vi "Driver Init.vi"(8 "error in (no error)":errorcluster, 11 "MSX-E3701 in":refnum<class "MSX-E3701.lvclass">) -> (0 "error out":errorcluster, 3 "MSX-E3701 out":refnum<class "MSX-E3701.lvclass">)   [LabVIEW 2014, in "MSX-E3701.lvlib" / "MSX-E3701.lvclass"]
doc: "Inicializa los valores recomendados por el datasheet del ADDI-DATA para iniciar la adquisición de datos en cualquiera de sus modos. Ademas inicia Los valores del Diagnostic, ganancia y offset."
uses:
  MSX-E3701.lvclass
  API/Typedef/Diagnostic Data.ctl
  MSX-E3701.lvclass/MSX-E3701.ctl
  DriverMasterSync/build/DriverMasterSync.lvlibp/Modules/HAL/DriverMasterSync/DriverMasterSyncClass/DriverMasterSync.lvclass
  API/MSX-E3701_dll.lvlib
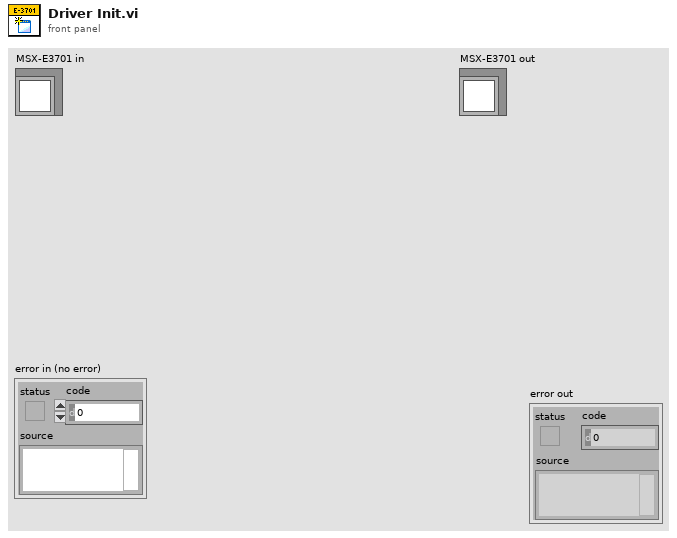
[diagram p1: front panel]
types:
  T1 = typedef "MSX-E3701_dll.lvlib/Diagnostic Data.ctl" = cluster{"Muestras Diag. Cycle":u32, "Tolerancia Cycle":sgl, "Tolerancia":sgl, "Mask Proteccion T":u64, "Promedio Transd":sgl[]}
  T2 = typedef "DriverMasterSync.lvlibp/HAL Config Data.ctl" = cluster{"HWSync Index":u32, "Driver Name":string, "Channel Mask":u64}
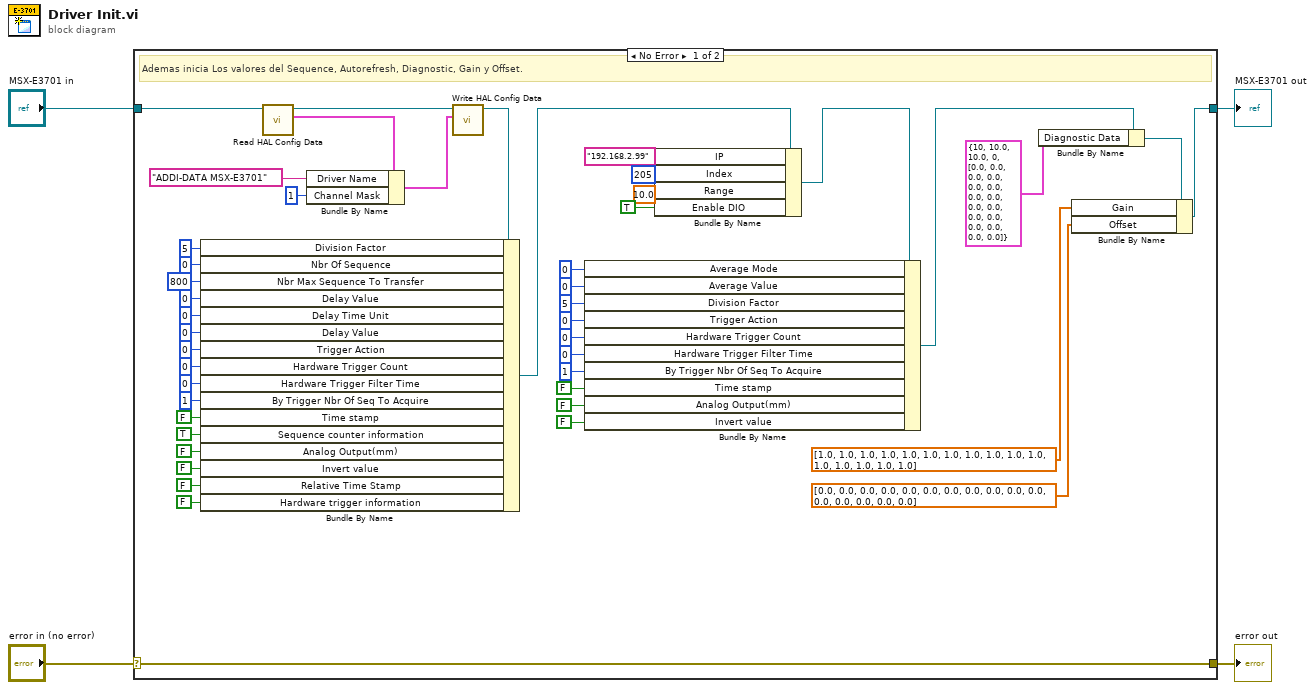
[diagram p0: block diagram]
diagram:
  n1 = case shown="No Error" "error in (no error)" {
    selector: "error in (no error)" -> [w50 w52]
    tunnel: [w50 w52] -> w3
    tunnel: [w16 w51] -> w1
    tunnel: "MSX-E3701 in" -> [w48 w51]
    frame No Error {
      # "Ademas inicia Los valores del Sequence, Autorefresh, Diagnostic, Gain y Offset."
      n2 = call "Read HAL Config Data.vi"("DriverMasterSync in"=w48) -> ("HAL Config Data"=w47:T2, "DriverMasterSync out"=w49:refnum<class "MSX-E3701.lvclass">)  [unwired: 8 in, 1 out]
      n3 = Bundle By Name(cluster=w47, "Driver Name"="ADDI-DATA MSX-E3701", "Channel Mask"=u64 1) -> (w46:T2)
      n4 = call "Write HAL Config Data.vi"("HAL Config Data"=w46, "DriverMasterSync in"=w49) -> ("DriverMasterSync out"=w44:refnum<class "MSX-E3701.lvclass">)  [unwired: 8 in, 1 out]
      n5 = Bundle By Name(cluster=w44, "Division Factor"=u64 5 ("Config Data.Sequence.Division Factor"), "Nbr Of Sequence"=u64 0 ("Config Data.Sequence.Nbr Of Sequence"), "Nbr Max Sequence To Transfer"=u64 800 ("Config Data.Sequence.Nbr Max Sequence To Transfer"), "Delay Value"=u64 0 ("Config Data.Sequence.Delay Mode"), "Delay Time Unit"=u64 0 ("Config Data.Sequence.Delay Time Unit"), "Delay Value"=u64 0 ("Config Data.Sequence.Delay Value"), "Trigger Action"=u64 0 ("Config Data.Sequence.Trigger Action"), "Hardware Trigger Count"=u64 0 ("Config Data.Sequence.Hardware Trigger Count"), "Hardware Trigger Filter Time"=u64 0 ("Config Data.Sequence.Hardware Trigger Filter Time"), "By Trigger Nbr Of Seq To Acquire"=u64 1 ("Config Data.Sequence.By Trigger Nbr Of Seq To Acquire"), "Time stamp"=FALSE ("Config Data.Sequence.Time stamp"), "Sequence counter information"=TRUE ("Config Data.Sequence.Sequence counter information"), "Analog Output(mm)"=FALSE ("Config Data.Sequence.Analog Output(mm)"), "Invert value"=FALSE ("Config Data.Sequence.Invert value"), "Relative Time Stamp"=FALSE ("Config Data.Sequence.Relative Time Stamp"), "Hardware trigger information"=FALSE ("Config Data.Sequence.Hardware trigger information")) -> (w13:refnum<class "MSX-E3701.lvclass">)
      n6 = Bundle By Name(cluster=w13, "IP"="192.168.2.99" ("Connection Data.IP"), "Index"=u64 205 ("Config Data.Index"), "Range"=sgl 10.0 ("Config Data.Range"), "Enable DIO"=TRUE ("Config Data.Enable DIO")) -> (w12:refnum<class "MSX-E3701.lvclass">)
      n7 = Bundle By Name(cluster=w12, "Average Mode"=u64 0 ("Config Data.Auto Refresh.Average Mode"), "Average Value"=u64 0 ("Config Data.Auto Refresh.Average Value"), "Division Factor"=u64 5 ("Config Data.Auto Refresh.Division Factor"), "Trigger Action"=u64 0 ("Config Data.Auto Refresh.Trigger Action"), "Hardware Trigger Count"=u64 0 ("Config Data.Auto Refresh.Hardware Trigger Count"), "Hardware Trigger Filter Time"=u64 0 ("Config Data.Auto Refresh.Hardware Trigger Filter Time"), "By Trigger Nbr Of Seq To Acquire"=u64 1 ("Config Data.Auto Refresh.By Trigger Nbr Of Seq To Acquire"), "Time stamp"=FALSE ("Config Data.Auto Refresh.Time stamp"), "Analog Output(mm)"=FALSE ("Config Data.Auto Refresh.Analog Output(mm)"), "Invert value"=FALSE ("Config Data.Auto Refresh.Invert value")) -> (w8:refnum<class "MSX-E3701.lvclass">)
      n8 = Bundle By Name(cluster=w8, "Diagnostic Data"=T1 {"Muestras Diag. Cycle"=10, "Tolerancia Cycle"=10.0, "Tolerancia"=10.0, "Mask Proteccion T"=0, "Promedio Transd"=[0.0, 0.0, 0.0, 0.0, 0.0, 0.0, 0.0, 0.0, 0.0, 0.0, 0.0, 0.0, 0.0, 0.0, 0.0, 0.0]}) -> (w7:refnum<class "MSX-E3701.lvclass">)
      n9 = Bundle By Name(cluster=w7, "Gain"=sgl[] [1.0, 1.0, 1.0, 1.0, 1.0, 1.0, 1.0, 1.0, 1.0, 1.0, 1.0, 1.0, 1.0, 1.0, 1.0, 1.0] ("Config Data.Gain"), "Offset"=sgl[] [0.0, 0.0, 0.0, 0.0, 0.0, 0.0, 0.0, 0.0, 0.0, 0.0, 0.0, 0.0, 0.0, 0.0, 0.0, 0.0] ("Config Data.Offset")) -> (w16:refnum<class "MSX-E3701.lvclass">)
    }
    frame Error {
    }
  }
  "error out" <- w3
  "MSX-E3701 out" <- w1
